vi "Allocate Channels.vi"(8 "error in":errorcluster, 11 "Num Channels":i32) -> (0 "error out":errorcluster, 3 "Num Channels Allocated":i32)   [LabVIEW 2015, in "LibSDL2_Mixer.lvlib"]
uses:
  LibSDL2_Mixer.lvlib
  LibSDL2 Wrapper/DLL/SDL2_mixer.dll
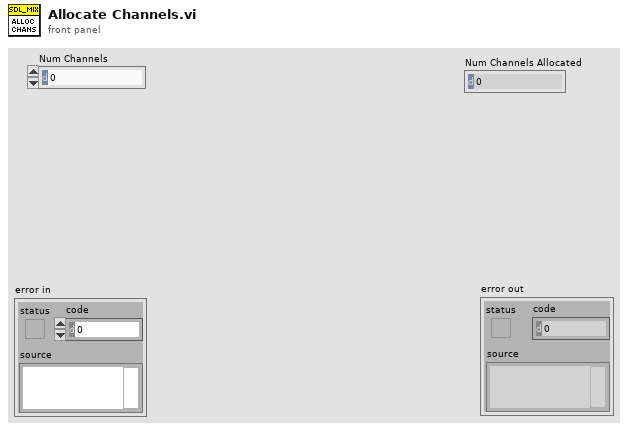
[diagram p1: front panel]
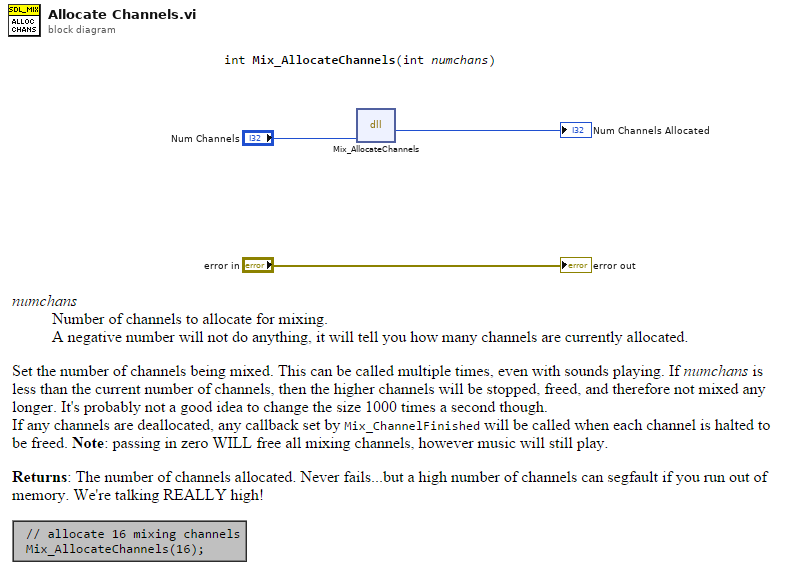
[diagram p0: block diagram]
diagram:
  n1 = dll-call lib="C:/dev/PGS/LabSDL2/Source/Libraries/LibSDL2 Wrapper/DLL/SDL2_mixer.dll" fn="Mix_AllocateChannels"("num channels"="Num Channels") -> ("return type"=→"Num Channels Allocated":i32)  [unwired: 4 in, 2 out]
  "error out" <- "error in"
